vi "NI Switch Get Relay Position.vi"(8 "error in (no error)":errorcluster, 10 "relay name":string, 11 "RelayOutput in":refnum<class "NISwitch.lvclass">) -> (0 "error out":errorcluster, 2 "position":T1=10 items=["Open"=10, "Closed"=11], 3 "RelayOutput out":refnum<class "NISwitch.lvclass">)   [LabVIEW 2023, in "HardwareAbstractionLayer_LVOOP.lvlib" / "NISwitch.lvclass"]
uses:
  NISwitch.lvclass
  <instrlib>/niSwitch/niSwitch.llb/niSwitch Relay Position.ctl
  NISwitch.lvclass/NISwitch.ctl
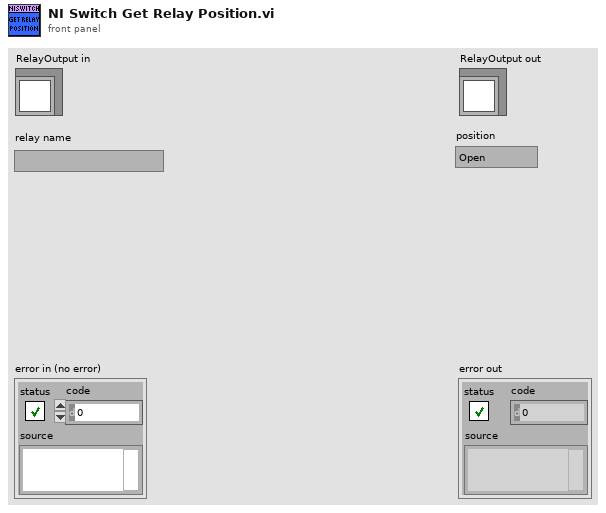
[diagram p1: front panel]
types:
  T1 = typedef "niSwitch Relay Position.ctl" = i32
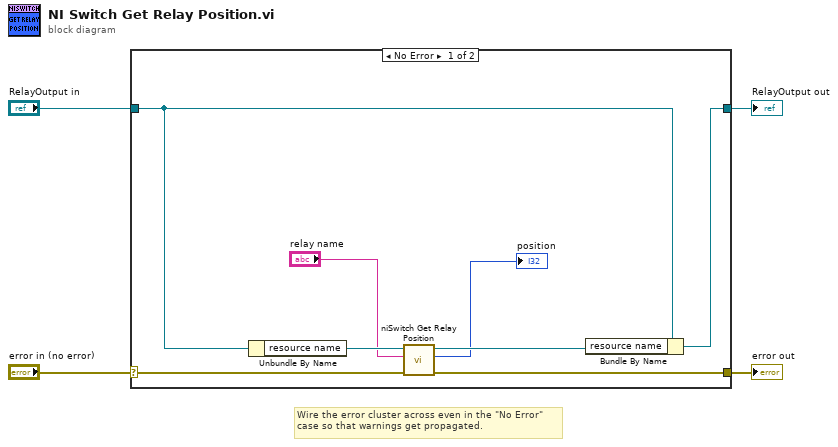
[diagram p0: block diagram]
diagram:
  # "Wire the error cluster across even in the \"No Error\"\ncase so that warnings get propagated."
  n1 = case shown="No Error" "error in (no error)" {
    selector: "error in (no error)" -> [w12 w14]
    tunnel: [w11 w14] -> w3
    tunnel: [w8 w13] -> w1
    tunnel: "RelayOutput in" -> [w9 w13]
    frame No Error {
      n2 = Unbundle By Name(w9) -> ("resource name"=w10:refnum<k15>)
      n3 = call <instrlib>:"niSwitch Get Relay Position.vi"("error in (no error)"=w12, "relay name"="relay name", "instrument handle"=w10) -> ("error out"=w11:errorcluster, "position"=→"position":T1, "instrument handle out"=w7:refnum<k15>)  [unwired: 6 in]
      n4 = Bundle By Name(cluster=w9, "resource name"=w7) -> (w8:refnum<class "NISwitch.lvclass">)
    }
    frame Error {
    }
  }
  "error out" <- w3
  "RelayOutput out" <- w1
